vi "Deserialize Mission Array.vi"(11 "Serialized Mission Array":string) -> (3 "Mission Object Array":refnum<class "Mission.lvclass">[](array[class]))   [LabVIEW 2011]
uses:
  Mission.lvclass
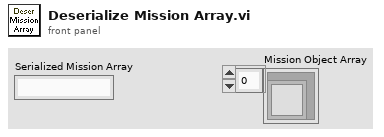
[diagram p1: front panel]
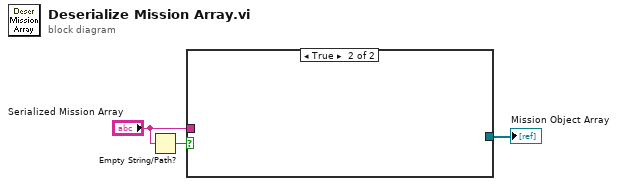
[diagram p0: block diagram]
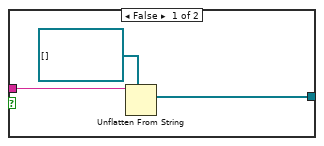
[diagram p2: hidden frame]
diagram:
  n1 = Empty String/Path?(string/path="Serialized Mission Array") -> (empty?=w2:bool)
  n2 = case shown="True" w2 {
    tunnel: [w6 _] -> w1
    tunnel: "Serialized Mission Array" -> [w5 _]
    frame False {
      n3 = Unflatten From String(type=refnum<class "Mission.lvclass">[] [] ("elements"), binary string=w5) -> (value=w6:refnum<class "Mission.lvclass">[])  [unwired: 3 in, 2 out]
    }
    frame True {
    }
  }
  "Mission Object Array" <- w1
